vi "Init.vi"(5 "PathControl.lvclass":refnum<class "PathControl.lvclass">, 6 "Environmental classes":refnum<class "Instrument.lvclass">[](array[class]), 7 "XML Handler.lvclass":refnum<class "XML Handler.lvclass">, 8 "error in (no error)":errorcluster, 9 "Instrumentes to Use":T1(array[cluster]), 10 "Device.lvclass":refnum<class "Device.lvclass">, 11 "IMD in":refnum<class "IMD.lvclass">) -> (0 "error out":errorcluster, 3 "IMD out":refnum<class "IMD.lvclass">)   [LabVIEW 2020, in "IMD.lvclass"]
doc: "Initializes the measurement.\nThis verifies that the instruments are present and adds them into the class data.\nIs also adds the xml handler into the class data."
uses:
  IMD.lvclass
  Devices/Device.lvclass
  Instruments/Instrument.lvclass
  XML Handler/XML Handler.lvclass
  Path Control/PathControl.lvclass
  Controls/Init states.ctl
  Instruments/Spectrum Analyzer/Spectrum Analyzer.lvclass
  Instruments/Signal Generator/Signal Generator.lvclass
  IMD.lvclass/IMD.ctl
  Instruments/Power Meter/Power Meter.lvclass
  Measurement.lvclass
panel:
  out "Current State":string
  out "Initializing IMD Measurement":u8(slide) scale=0.0..100.0
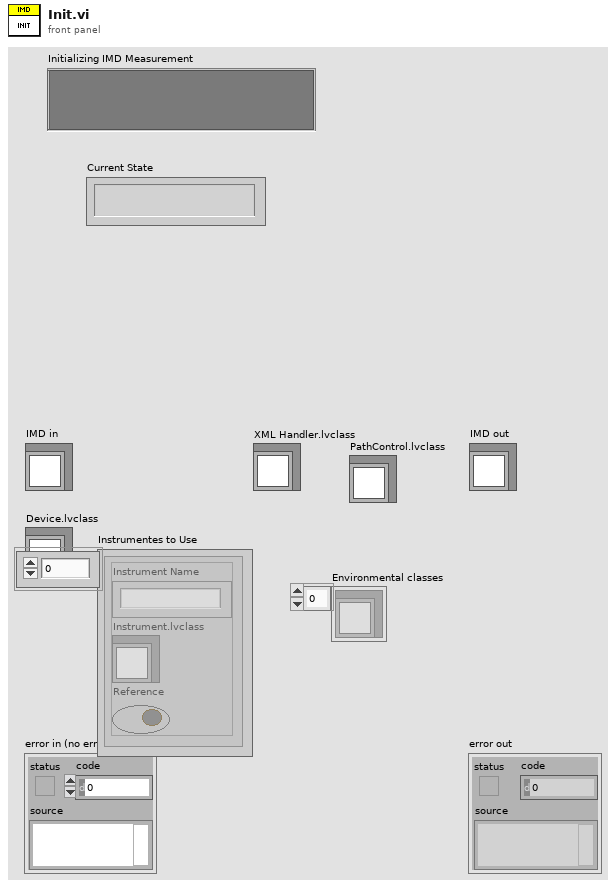
[diagram p1: front panel]
types:
  T1 = cluster{"Instrument Name":string, "Instrument.lvclass":refnum<class "Instrument.lvclass">, "Reference":bool}[]
  T2 = typedef "IMD.lvclass/Init states.ctl" = enum16{"Verify instruments", "Init Parameters", "Init Instruments", "Done"}
  T3 = typedef "IMD.lvclass/Config info.ctl" = cluster{"RBW":dbl, "VBW ":dbl, "Number of Averages":dbl, "Average On":bool, "Frequency (MHz)":string, "Offset Frequency (MHz)":string, "Power (dBm)":string, "Delta Power (dB)":string, "Uneven IMD":bool, "Loop order":T4, "Stop level":dbl, "IMD2":bool, "IMD3":bool}
  T4 = typedef "IMD.lvclass/Loop order.ctl" = enum16{"Device -> Power -> Frequency -> Offset", "Device -> Frequency -> Power -> Offset"}
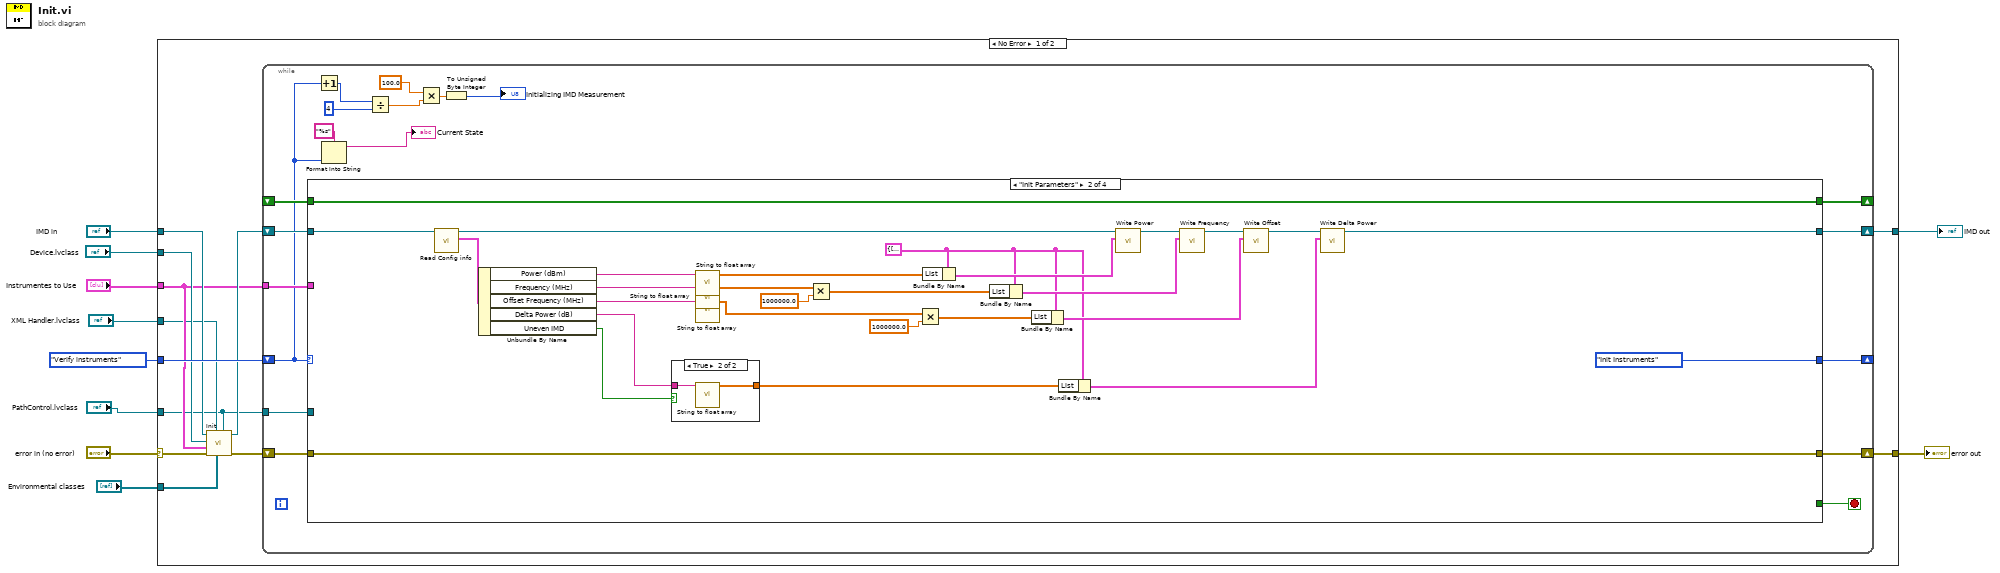
[diagram p0: block diagram]
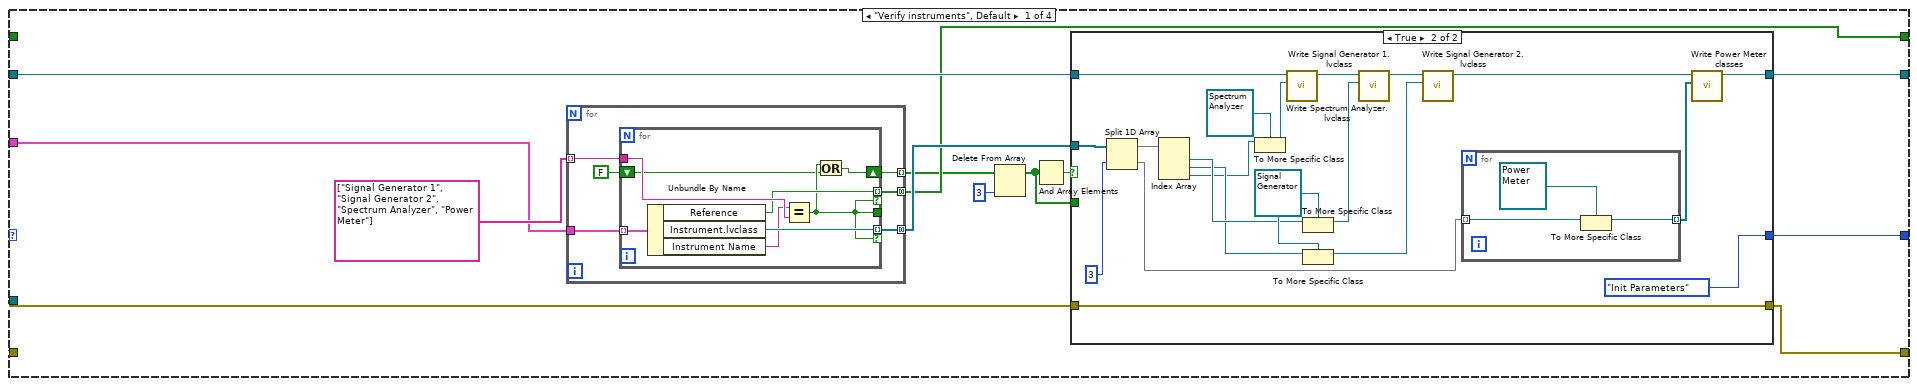
[diagram p2: hidden frame]
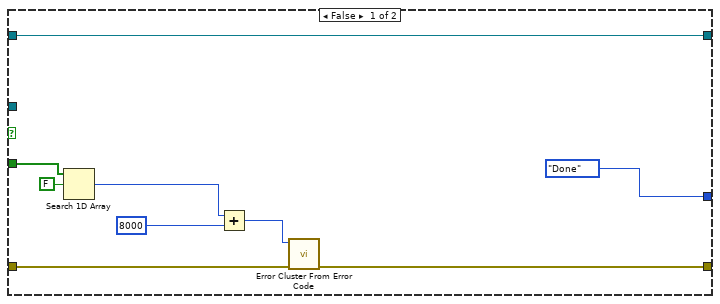
[diagram p3: hidden frame]
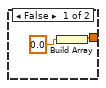
[diagram p4: hidden frame]
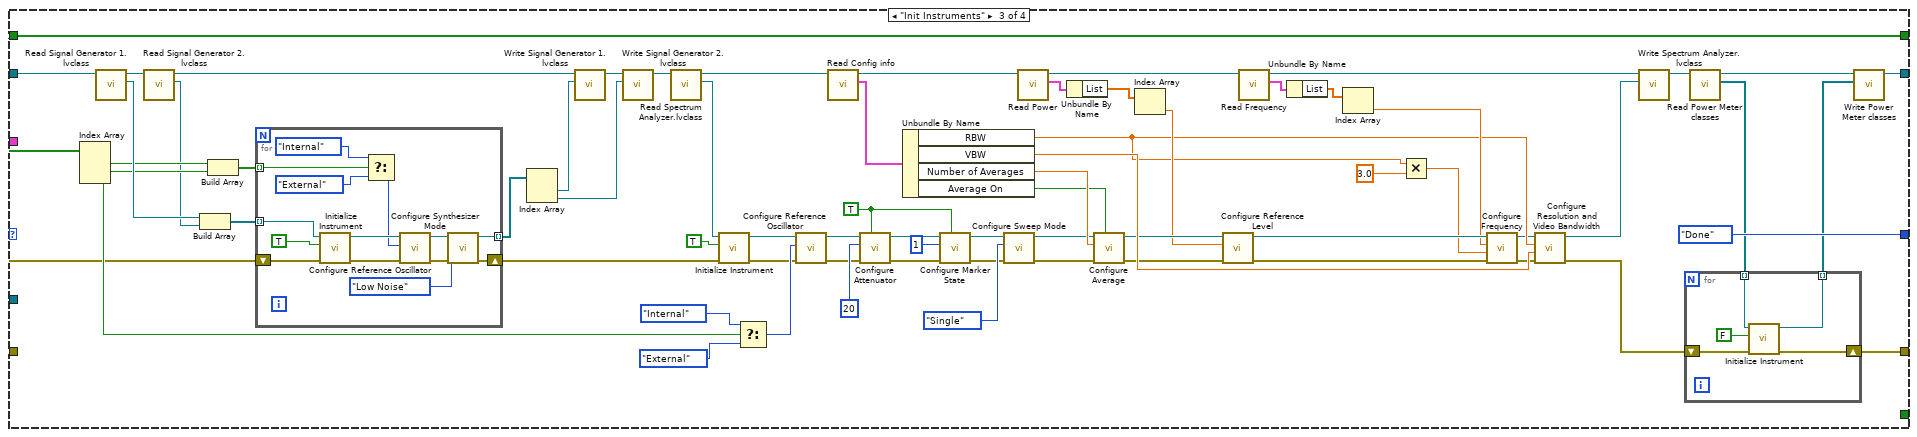
[diagram p5: hidden frame]
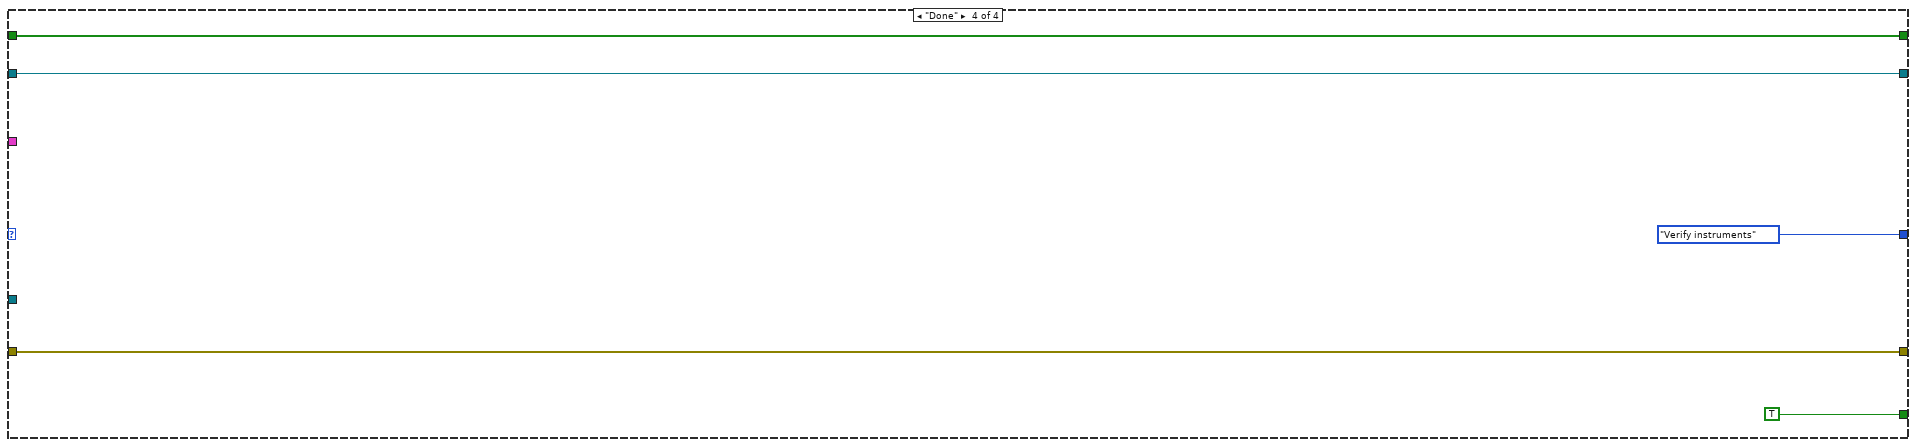
[diagram p6: hidden frame]
diagram:
  n1 = case shown="No Error" "error in (no error)" {
    selector: "error in (no error)" -> [w19 w226]
    tunnel: "Instrumentes to Use" -> [w13 _]
    tunnel: "Device.lvclass" -> [w14 _]
    tunnel: "IMD in" -> [w17 w227]
    tunnel: Init_states."Verify instruments" -> [w20 _]
    tunnel: [w22 w226] -> w5
    tunnel: [w21 w227] -> w4
    tunnel: "XML Handler.lvclass" -> [w12 _]
    tunnel: "Environmental classes" -> [w15 _]
    tunnel: "PathControl.lvclass" -> [w11 _]
    frame No Error {
      n2 = call-parent "Init.vi"("PathControl.lvclass"=w11, "Environmental classes"=w15, "XML Handler.lvclass"=w12, "error in (no error)"=w19, "Instruments to Use"=w13, "Device.lvclass"=w14, "Measurements in"=w17) -> ("error out"=w18:errorcluster, "Measurements out"=w16:refnum<class "IMD.lvclass">)  [unwired: 3 in]
      n3 = while {
        shift-right: [w37] -> w22
        shift-left: w18 -> [w38]
        tunnel: w13 -> [w41]
        shift-right: [w39] -> w21
        shift-left: w16 -> [w40]
        shift-right: [w35] -> _
        shift-left: w20 -> [w24]
        shift-right: [w34] -> _
        shift-left: _ -> [w33]
        tunnel: w11 -> [w23]
        stop <- w36 stop-if-true
        n4 = case shown="\"Init Parameters\"" w24 {
          tunnel: w41 -> [w48 _ _ _]
          tunnel: w40 -> [w50 w126 w143 w221]
          tunnel: [w54 w112 w136 w221] -> w39
          tunnel: w38 -> [w53 w127 w144 w223]
          tunnel: [w52 w127 w141 w223] -> w37
          tunnel: [w51 Init_states."Init Instruments" Init_states."Done" Init_states."Verify instruments"] -> w35
          tunnel: [_ _ _ TRUE] -> w36
          tunnel: [w46 w118 w183 w225] -> w34
          tunnel: w33 -> [_ w118 w183 w225]
          tunnel: w23 -> [_ _ _ _]
          frame "Verify instruments", Default {
            n5 = for {
              tunnel: [w60] -> w47 mode=concatenating
              tunnel: [w55] -> w45 mode=indexing
              tunnel: [w59] -> w46 mode=concatenating
              tunnel: string[] ["Signal Generator 1", "Signal Generator 2", "Spectrum Analyzer", "Power Meter"] -> [w58] mode=indexing
              tunnel: w48 -> [w57]
              n6 = for {
                tunnel: w57 -> [w65] mode=indexing
                tunnel: w58 -> [w68]
                tunnel: [w67] -> w60 mode=indexing if=w62
                tunnel: [w62] -> _
                tunnel: [w66] -> w59 mode=indexing if=w62
                shift-right: [w63] -> w55
                shift-left: FALSE -> [w61]
                n7 = Unbundle By Name(w65) -> ("Reference"=w66:bool, "Instrument.lvclass"=w67:refnum<class "Instrument.lvclass">, "Instrument Name"=w64:string)
                n8 = Equal?(x=w64, y=w68) -> (x = y?=w62:bool)
                n9 = Or(x=w62, y=w61) -> (x .or. y?=w63:bool)
              }
            }
            n10 = Delete From Array(array=w45, index=3) -> (array with subset deleted=w42:bool[])  [unwired: 1 in, 1 out]
            n11 = And Array Elements(Boolean array=w42) -> (logical AND=w43:bool)
            n12 = case shown="True" w43 {
              tunnel: w47 -> [_ w82]
              tunnel: w50 -> [w77 w97]
              tunnel: [w77 w84] -> w54
              tunnel: w53 -> [w76 w91]
              tunnel: [w73 w91] -> w52
              tunnel: [Init_states."Done" Init_states."Init Parameters"] -> w51
              tunnel: w42 -> [w70 _]
              frame False {
                n13 = Search 1D Array(1D array=w70, element=FALSE) -> (index of element=w69:i32)  [unwired: 1 in]
                n14 = Add(x=w69, y=8000) -> (x+y=w74:i32)
                n15 = call <vilib>:"Error Cluster From Error Code.vi"("error in (no error)"=w76, "error code (0)"=w74) -> ("error out"=w73:errorcluster)  [unwired: 7 in]
              }
              frame True {
                w90 = refnum<class "Signal Generator.lvclass"> refnum ("Signal Generator.lvclass")
                n16 = Split 1D Array(array=w82, index=3) -> (first subarray=w80:refnum<class "Instrument.lvclass">[], second subarray=w79:refnum<class "Instrument.lvclass">[])
                n17 = Index Array(array=w80) -> (element #1=w87:refnum<class "Instrument.lvclass">, element #2=w86:refnum<class "Instrument.lvclass">, element #3=w85:refnum<class "Instrument.lvclass">)  [unwired: 3 in]
                n18 = To More Specific Class(target class=refnum<class "Spectrum Analyzer.lvclass"> refnum ("Spectrum Analyzer.lvclass"), reference=w85) -> (specific class reference=w95:refnum<class "Spectrum Analyzer.lvclass">)  [unwired: 1 in, 1 out]
                n19 = call "Write Spectrum Analyzer.lvclass.vi"("Spectrum Analyzer.lvclass"=w95, "IMD in"=w97) -> ("IMD out"=w96:refnum<class "IMD.lvclass">)  [unwired: 9 in]
                n20 = To More Specific Class(target class=w90, reference=w87) -> (specific class reference=w93:refnum<class "Signal Generator.lvclass">)  [unwired: 1 in, 1 out]
                n21 = To More Specific Class(target class=w90, reference=w86) -> (specific class reference=w88:refnum<class "Signal Generator.lvclass">)  [unwired: 1 in, 1 out]
                n22 = call "Write Signal Generator 1.lvclass.vi"("Signal Generator 1.lvclass"=w93, "IMD in"=w96) -> ("IMD out"=w89:refnum<class "IMD.lvclass">)  [unwired: 9 in]
                n23 = call "Write Signal Generator 2.lvclass.vi"("Signal Generator.lvclass"=w88, "IMD in"=w89) -> ("IMD out"=w78:refnum<class "IMD.lvclass">)  [unwired: 9 in]
                n24 = for {
                  tunnel: [w99] -> w83 mode=indexing
                  tunnel: w79 -> [w98] mode=indexing
                  n25 = To More Specific Class(target class=refnum<class "Power Meter.lvclass"> refnum ("Power Meter.lvclass"), reference=w98) -> (specific class reference=w99:refnum<class "Power Meter.lvclass">)  [unwired: 1 in, 1 out]
                }
                n26 = call-dynamic "Write Power Meter classes.vi"("Power Meter classes"=w83, "IMD in"=w78) -> ("IMD out"=w84:refnum<class "IMD.lvclass">)  [unwired: 9 in]
              }
            }
          }
          frame "Init Parameters" {
            w114 = cluster{"List":dbl[], "Index":i32, "Last":bool} {"List"=[], "Index"=0, "Last"=FALSE} ("Power")
            n27 = call "Read Config info.vi"("IMD in"=w126) -> ("Config info"=w125:T3, "IMD out"=w124:refnum<class "IMD.lvclass">)  [unwired: 9 in]
            n28 = Unbundle By Name(w125) -> ("Power (dBm)"=w109:string, "Frequency (MHz)"=w107:string, "Offset Frequency (MHz)"=w108:string, "Delta Power (dB)"=w116:string, "Uneven IMD"=w117:bool)
            n29 = case shown="True" w117 {
              tunnel: w116 -> [_ w132]
              tunnel: [w129 w131] -> w115
              frame False {
                n30 = Build Array(0.0) -> (w129:dbl[])
              }
              frame True {
                n31 = call "String to float array.vi"("String"=w132) -> ("Array - Numeric"=w131:dbl[])  [unwired: 9 in, 1 out]
              }
            }
            n32 = call "String to float array.vi"("String"=w109) -> ("Array - Numeric"=w110:dbl[])  [unwired: 9 in, 1 out]
            n33 = call "String to float array.vi"("String"=w107) -> ("Array - Numeric"=w102:dbl[])  [unwired: 9 in, 1 out]
            n34 = call "String to float array.vi"("String"=w108) -> ("Array - Numeric"=w104:dbl[])  [unwired: 9 in, 1 out]
            n35 = Multiply(x=w102, y=1000000.0) -> (x*y=w101:dbl[])
            n36 = Multiply(x=w104, y=1000000.0) -> (x*y=w103:dbl[])
            n37 = Bundle By Name(cluster=w114, "List"=w110) -> (w122:cluster{"List":dbl[], "Index":i32, "Last":bool})
            n38 = Bundle By Name(cluster=w114, "List"=w101) -> (w121:cluster{"List":dbl[], "Index":i32, "Last":bool})
            n39 = Bundle By Name(cluster=w114, "List"=w103) -> (w119:cluster{"List":dbl[], "Index":i32, "Last":bool})
            n40 = Bundle By Name(cluster=w114, "List"=w115) -> (w111:cluster{"List":dbl[], "Index":i32, "Last":bool})
            n41 = call "Write Power.vi"("Power"=w122, "IMD in"=w124) -> ("IMD out"=w123:refnum<class "IMD.lvclass">)  [unwired: 9 in]
            n42 = call "Write Frequency.vi"("Frequency"=w121, "IMD in"=w123) -> ("IMD out"=w120:refnum<class "IMD.lvclass">)  [unwired: 9 in]
            n43 = call "Write Offset.vi"("Offset"=w119, "IMD in"=w120) -> ("IMD out"=w113:refnum<class "IMD.lvclass">)  [unwired: 9 in]
            n44 = call "Write Delta Power.vi"("Delta Power"=w111, "IMD in"=w113) -> ("IMD out"=w112:refnum<class "IMD.lvclass">)  [unwired: 9 in]
          }
          frame "Init Instruments" {
            w189 = TRUE ("Auto Attenuator (T)")
            n45 = Index Array(array=w183) -> (element #1=w182:bool, element #2=w179:bool, element #3=w163:bool)  [unwired: 3 in]
            n46 = call "Read Signal Generator 1.lvclass.vi"("IMD in"=w143) -> ("Signal Generator 1.lvclass"=w201:refnum<class "Signal Generator.lvclass">, "IMD out"=w181:refnum<class "IMD.lvclass">)  [unwired: 9 in]
            n47 = call "Read Signal Generator 2.lvclass.vi"("IMD in"=w181) -> ("Signal Generator.lvclass"=w177:refnum<class "Signal Generator.lvclass">, "IMD out"=w175:refnum<class "IMD.lvclass">)  [unwired: 9 in]
            n48 = Build Array(w201, w177) -> (w178:refnum<class "Signal Generator.lvclass">[])
            n49 = Build Array(w182, w179) -> (w180:bool[])
            n50 = for {
              tunnel: w178 -> [w220] mode=indexing
              tunnel: w180 -> [w212] mode=indexing
              shift-right: [w208] -> w176
              shift-left: w144 -> [w218]
              tunnel: [w207] -> w173 mode=indexing
              n51 = call-dynamic "Initialize Instrument.vi"("error in (no error)"=w218, "Reset"=TRUE, "Instrument in"=w220) -> ("error out"=w217:errorcluster, "Instrument out"=w216:refnum<class "Signal Generator.lvclass">)  [unwired: 7 in]
              n52 = Select(t=enum16{"Internal", "External"}."Internal" ("Reference Mode"), s=w212, f=enum16{"Internal", "External"}."External") -> (s? t:f=w210:enum16{"Internal", "External"})
              n53 = call-dynamic "Configure Reference Oscillator.vi"("error in (no error)"=w217, "Reference Mode"=w210, "Signal Generator in"=w216) -> ("error out"=w214:errorcluster, "Signal Generator out"=w215:refnum<class "Signal Generator.lvclass">)  [unwired: 7 in]
              n54 = call-dynamic "Configure Synthesizer Mode.vi"("error in (no error)"=w214, "Synthesizer Mode"=enum16{"Normal", "Low Noise"}."Low Noise", "Signal Generator in"=w215) -> ("error out"=w208:errorcluster, "Signal Generator out"=w207:refnum<class "Signal Generator.lvclass">)  [unwired: 7 in]
            }
            n55 = Index Array(array=w173) -> (element #1=w172:refnum<class "Signal Generator.lvclass">, element #2=w171:refnum<class "Signal Generator.lvclass">)  [unwired: 2 in]
            n56 = call "Write Signal Generator 1.lvclass.vi"("Signal Generator 1.lvclass"=w172, "IMD in"=w175) -> ("IMD out"=w174:refnum<class "IMD.lvclass">)  [unwired: 9 in]
            n57 = call "Write Signal Generator 2.lvclass.vi"("Signal Generator.lvclass"=w171, "IMD in"=w174) -> ("IMD out"=w184:refnum<class "IMD.lvclass">)  [unwired: 9 in]
            n58 = call "Read Spectrum Analyzer.lvclass.vi"("IMD in"=w184) -> ("Spectrum Analyzer.lvclass"=w200:refnum<class "Spectrum Analyzer.lvclass">, "IMD out"=w196:refnum<class "IMD.lvclass">)  [unwired: 9 in]
            n59 = call-dynamic "Initialize Instrument.vi"("error in (no error)"=w176, "Reset"=TRUE, "Instrument in"=w200) -> ("error out"=w166:errorcluster, "Instrument out"=w168:refnum<class "Spectrum Analyzer.lvclass">)  [unwired: 7 in]
            n60 = Select(t=enum16{"Internal", "External"}."Internal" ("Reference Mode"), s=w163, f=enum16{"Internal", "External"}."External") -> (s? t:f=w167:enum16{"Internal", "External"})
            n61 = call-dynamic "Configure Reference Oscillator.vi"("error in (no error)"=w166, "Reference Oscillator (Internal)"=w167, "Spectrum Analyzer in"=w168) -> ("error out"=w165:errorcluster, "Spectrum Analyzer out"=w164:refnum<class "Spectrum Analyzer.lvclass">)  [unwired: 7 in]
            n62 = call "Read Config info.vi"("IMD in"=w196) -> ("Config info"=w195:T3, "IMD out"=w135:refnum<class "IMD.lvclass">)  [unwired: 9 in]
            n63 = call-dynamic "Configure Attenuator.vi"("Auto Attenuator (T)"=w189, "error in (no error)"=w165, "Attenuator (dB)"=u32 20, "Spectrum Analyzer in"=w164) -> ("error out"=w191:errorcluster, "Spectrum Analyzer out"=w190:refnum<class "Spectrum Analyzer.lvclass">)  [unwired: 6 in]
            n64 = Unbundle By Name(w195) -> ("RBW"=w152:dbl, "VBW"=w194:dbl, "Number of Averages"=w193:dbl, "Average On"=w192:bool)
            n65 = call-dynamic "Configure Marker State.vi"("Maker On (F)"=w189, "error in (no error)"=w191, "Marker Number (1)"=u32 1, "Spectrum Analyzer in"=w190) -> ("error out"=w185:errorcluster, "Spectrum Analyzer out"=w186:refnum<class "Spectrum Analyzer.lvclass">)  [unwired: 6 in]
            n66 = call-dynamic "Configure Sweep Mode.vi"("error in (no error)"=w185, "Sweep Mode"=enum16{"Continuous", "Single"}."Single", "Spectrum Analyzer in"=w186) -> ("error out"=w146:errorcluster, "Spectrum Analyzer out"=w145:refnum<class "Spectrum Analyzer.lvclass">)  [unwired: 7 in]
            n67 = call "Read Power.vi"("IMD in"=w135) -> ("Power"=w162:cluster{"List":dbl[], "Index":i32, "Last":bool}, "IMD out"=w133:refnum<class "IMD.lvclass">)  [unwired: 9 in]
            n68 = Unbundle By Name(w162) -> ("List"=w159:dbl[])
            n69 = call-dynamic "Configure Average.vi"("Average On (F)"=w192, "error in (no error)"=w146, "Average"=w193, "Spectrum Analyzer in"=w145) -> ("error out"=w157:errorcluster, "Spectrum Analyzer out"=w160:refnum<class "Spectrum Analyzer.lvclass">)  [unwired: 6 in]
            n70 = Index Array(array=w159) -> (element=w158:dbl)  [unwired: 1 in]
            n71 = call-dynamic "Configure Reference Level.vi"("error in (no error)"=w157, "Reference Level [dBm]"=w158, "Spectrum Analyzer in"=w160) -> ("error out"=w154:errorcluster, "Spectrum Analyzer out"=w155:refnum<class "Spectrum Analyzer.lvclass">)  [unwired: 7 in]
            n72 = call "Read Frequency.vi"("IMD in"=w133) -> ("Frequency"=w161:cluster{"List":dbl[], "Index":i32, "Last":bool}, "IMD out"=w134:refnum<class "IMD.lvclass">)  [unwired: 9 in]
            n73 = Unbundle By Name(w161) -> ("List"=w156:dbl[])
            n74 = Index Array(array=w156) -> (element=w153:dbl)  [unwired: 1 in]
            n75 = Multiply(x=w152, y=3.0) -> (x*y=w150:dbl)
            n76 = call-dynamic "Configure Frequency.vi"("error in (no error)"=w154, "Span/Stop Frequency [Hz]"=w150, "Center/Start Frequency [Hz]"=w153, "Spectrum Analyzer in"=w155) -> ("error out"=w148:errorcluster, "Spectrum Analyzer out"=w149:refnum<class "Spectrum Analyzer.lvclass">)  [unwired: 6 in]
            n77 = call-dynamic "Configure Resolution and Video Bandwidth.vi"("error in (no error)"=w148, "VBW [Hz]"=w194, "RBW [Hz]"=w152, "Spectrum Analyzer in"=w149) -> ("error out"=w142:errorcluster, "Spectrum Analyzer out"=w147:refnum<class "Spectrum Analyzer.lvclass">)  [unwired: 6 in]
            n78 = call "Write Spectrum Analyzer.lvclass.vi"("Spectrum Analyzer.lvclass"=w147, "IMD in"=w134) -> ("IMD out"=w137:refnum<class "IMD.lvclass">)  [unwired: 9 in]
            n79 = call-dynamic "Read Power Meter classes.vi"("IMD in"=w137) -> ("Power Meter classes"=w139:refnum<class "Power Meter.lvclass">[], "IMD out"=w138:refnum<class "IMD.lvclass">)  [unwired: 9 in]
            n80 = for {
              tunnel: w139 -> [w205] mode=indexing
              tunnel: [w202] -> w140 mode=indexing
              shift-right: [w203] -> w141
              shift-left: w142 -> [w206]
              n81 = call-dynamic "Initialize Instrument.vi"("error in (no error)"=w206, "Reset"=FALSE, "Instrument in"=w205) -> ("error out"=w203:errorcluster, "Instrument out"=w202:refnum<class "Power Meter.lvclass">)  [unwired: 7 in]
            }
            n82 = call-dynamic "Write Power Meter classes.vi"("Power Meter classes"=w140, "IMD in"=w138) -> ("IMD out"=w136:refnum<class "IMD.lvclass">)  [unwired: 9 in]
          }
          frame "Done" {
          }
        }
        n83 = Increment(x=w24) -> (x+1=w31:T2)
        n84 = Format Into String(format string="%s", w24) -> (resulting string=→"Current State":string)  [unwired: 2 in, 1 out]
        n85 = Divide(x=w31, y=4) -> (x/y=w29:dbl)
        n86 = Multiply(x=100.0 ("y"), y=w29) -> (x*y=w27:dbl)
        n87 = To Unsigned Byte Integer(number=w27) -> (unsigned 8bit integer=→"Initializing IMD Measurement":u8)
      }
    }
    frame Error {
    }
  }
  "error out" <- w5
  "IMD out" <- w4
